vi "Populating the Asynchronous Call Pool.vi"() -> ()   [LabVIEW 2020]
doc: "<b>Example Description</b>\n\nThis example shows the difference in performance between pre-populating the asynchronous call pool or not. Pre-populating the pool will prevent the Start Asynchronous Call node from needing to switch to the LabVIEW UI thread and create a data space.\n\nWhen running this example, you can see the time it takes to start asynchronous calls is less when the asynchronous call pool was properly pre-populated.\n\n<b>Overview of Asynchronous Call Pool</b>\n\nWhen performing asynchronous calls, an asynchronous call pool of data spaces is automatically created by the Open VI Reference function. By default, the call pool will be sized based on the number of computer cores.\n\nWhen the Start Asynchronous Call node is called, it will attempt to retrieve a data space from the asynchronous call pool. If there are no data spaces available, the Start Asynchronous Call node will automatically create a data space on demand and add it to the pool. This data space creation must be done in the LabVIEW UI thread. The Start Asynchronous Call node will only require the UI thread when it needs to create a data space.\n\nData spaces are automatically returned to the asynchronous call pool differently depending on whether you are performing a call and collect or a call and forget. For the call and collect use case, this is done only after the Wait On Asynchronous Call completes and results have been collected. For the call and forget use case, this is done as soon as the target VI execution completes.\n\nBecause the Start Asynchronous call node can add data spaces to the pool on demand, this can cause short delays when starting a call. These delays can be avoided by using the Populate Asynchronous Call Pool method to create data spaces beforehand."
panel:
  in  "Number of calls":i32=100
  out "Auto Allocate Pool -- Time to start all calls (ms)":u32[](array[numeric])
  out "Preallocate Pool -- Time to start all calls (ms)":u32[](array[numeric])
  # "Overview: Demonstrates the use of the  Populate Asynchronous Call Pool method with Asynchronous VI Calls.\nInstructions:\nRun the VI. Observe the benchmark values below. See the block diagram for more information."
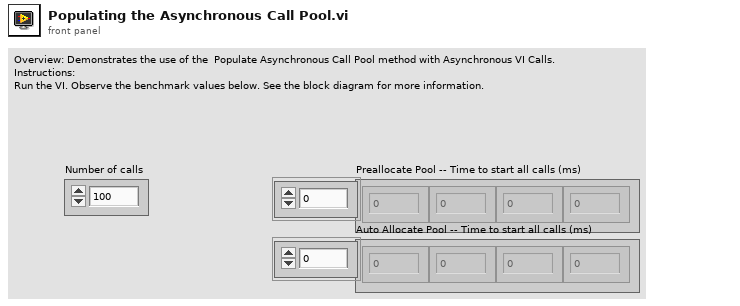
[diagram p1: front panel]
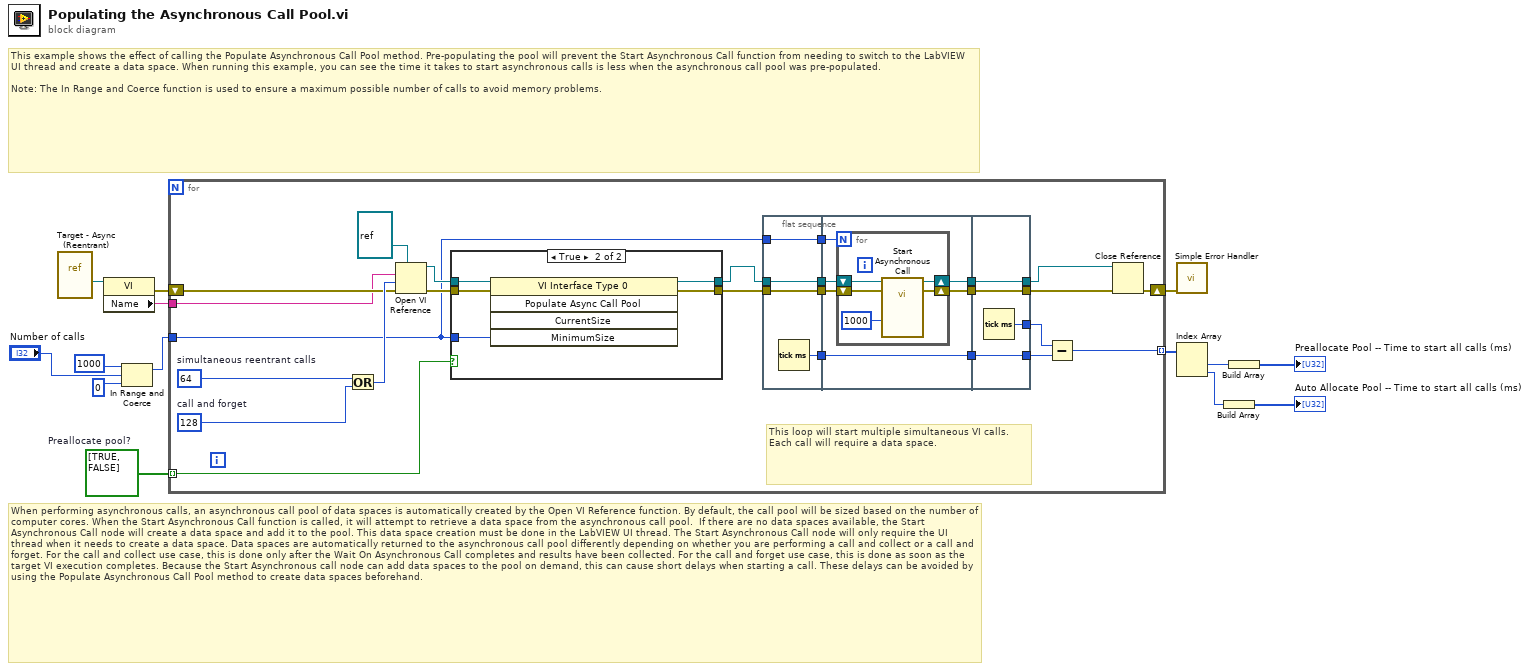
[diagram p0: block diagram]
diagram:
  w14 = bool[] [TRUE, FALSE]  # Preallocate pool?
  # "When performing asynchronous calls, an asynchronous call pool of data spaces is automatically created by the Open VI Reference function. By default, the call pool will be sized based on the number of computer cores. When the Start Asynchronous Call function is called, it will attempt to retrieve a data space from the asynchronous call pool.  If there are no data spaces available, the Start Asynchronous Call node will create a data space and add it to the pool. This data space creation must be done in the LabVIEW UI thread. The Start Asynchronous Call node will only require the UI thread when it needs to create a data space. Data spaces are automatically returned to the asynchronous call pool differently depending on whether you are performing a call and collect or a call and forget. For the call and collect use case, this is done only after the Wait On Asynchronous Call completes and results have been collected. For the call and forget use case, this is done as soon as the target VI execution completes. Because the Start Asynchronous call node can add data spaces to the pool on demand, this can cause short delays when starting a call. These delays can be avoided by using the Populate Asynchronous Call Pool method to create data spaces beforehand."
  # "This example shows the effect of calling the Populate Asynchronous Call Pool method. Pre-populating the pool will prevent the Start Asynchronous Call function from needing to switch to the LabVIEW UI thread and create a data space. When running this example, you can see the time it takes to start asynchronous calls is less when the asynchronous call pool was pre-populated.\n\nNote: The In Range and Coerce function is used to ensure a maximum possible number of calls to avoid memory problems."
  n1 = vi-ref "Target - Async (Reentrant).vi"() -> (w5:refnum<vi>)
  n2 = property class="VI"(reference=w5) -> (error out=w4:errorcluster, "Name"=w3:string)  [unwired: 1 in, 1 out]
  n3 = In Range and Coerce(upper limit=1000 ("y"), x="Number of calls", lower limit=0) -> (coerced(x)=w8:i32)  [unwired: 1 out]
  n4 = for {
    tunnel: [w29] -> w13 mode=indexing
    tunnel: w14 -> [w28] mode=indexing
    tunnel: w8 -> [w27]
    shift-right: [w36] -> w6
    shift-left: w4 -> [w25]
    tunnel: w3 -> [w24]
    w26 = 64  # simultaneous reentrant calls
    w35 = 128  # call and forget
    # "This loop will start multiple simultaneous VI calls. Each call will require a data space."
    n5 = Or(x=w26, y=w35) -> (x .or. y?=w34:i32)
    n6 = Open VI Reference(type specifier VI Refnum (for type only)=refnum<vi> refnum, vi path=w24, options=w34, error in (no error)=w25) -> (vi reference=w33:refnum<vi>, error out=w32:errorcluster)  [unwired: 2 in]
    n7 = case shown="True" w28 {
      tunnel: w33 -> [w60 w65]
      tunnel: w32 -> [w59 w64]
      tunnel: [w60 w63] -> w31
      tunnel: [w59 w62] -> w30
      tunnel: w27 -> [_ w61]
      frame False {
      }
      frame True {
        n8 = invoke class="VI Interface Type 0" method="Populate Async Call Pool"(reference=w65, error in=w64, "MinimumSize"=w61) -> (reference out=w63:refnum<vi>, error out=w62:errorcluster)  [unwired: 2 in, 3 out]
      }
    }
    n9 = flat-sequence {
      tunnel: w30 -> [w42]
      tunnel: w31 -> [w43]
      tunnel: [w43] -> w23
      tunnel: [w42] -> w22
      tunnel: [w41] -> w21
      tunnel: w27 -> [w40]
      tunnel: [w40] -> w20
      tunnel: [w49] -> w19
      tunnel: [w48] -> w18
      tunnel: w23 -> [w47]
      tunnel: w22 -> [w46]
      tunnel: [w45] -> w17
      tunnel: w21 -> [w45]
      tunnel: w20 -> [w44]
      tunnel: [w57] -> w37
      tunnel: [w58] -> w38
      tunnel: w19 -> [w58]
      tunnel: w18 -> [w57]
      tunnel: [w56] -> w16
      tunnel: [w55] -> w15
      tunnel: w17 -> [w55]
      frame #0 {
        n10 = Tick Count (ms)() -> (millisecond timer value=w41:u32)
      }
      frame #1 {
        n11 = for {
          N: w44 -> [_]
          shift-right: [w54] -> w49
          shift-left: w46 -> [w51]
          shift-right: [w53] -> w48
          shift-left: w47 -> [w52]
          n12 = call-by-ref "Start Asynchronous Call"(reference=w52, error in=w51, "Wait (Milliseconds)"=u32 1000) -> (reference out=w53:refnum<vi>, error out=w54:errorcluster)  [unwired: 10 in, 1 out]
        }
      }
      frame #2 {
        n13 = Tick Count (ms)() -> (millisecond timer value=w56:u32)
      }
    }
    n14 = Subtract(x=w16, y=w15) -> (x-y=w29:u32)
    n15 = Close Reference(reference=w37, error in (no error)=w38) -> (error out=w36:errorcluster)
  }
  n16 = call <vilib>:"Simple Error Handler.vi"("error in (no error)"=w6) -> ()  [unwired: 4 in, 5 out]
  n17 = Index Array(array=w13) -> (element #1=w12:u32, element #2=w7:u32)  [unwired: 2 in]
  n18 = Build Array(w7) -> (→"Auto Allocate Pool -- Time to start all calls (ms)":u32[])
  n19 = Build Array(w12) -> (→"Preallocate Pool -- Time to start all calls (ms)":u32[])
